vi "createSoundWave.vi"(7 "Device ID":u32, 8 "error in (no error)":errorcluster, 9 "duration (s)":dbl, 10 "frequency":dbl=10.0 format="%0.2p", 11 "Volume":dbl(slide)=50.0 scale=0.0..100.0) -> (0 "error out":errorcluster, 3 "Sound out":refnum<class "Sound.lvclass">)   [LabVIEW 2019, in "Sound.lvclass"]
uses:
  Sound.lvclass
  <vilib>/sound2/lvsound2.llb/Sampling Mode.ctl
  <vilib>/sound2/lvsound2.llb/Sound Data Format.ctl
  Sound.lvclass/Sound.ctl
  <vilib>/sound2/lvsound2.llb/Sound Output Set Volume (Single).vi
  <vilib>/measure/NI_MABase.lvlib
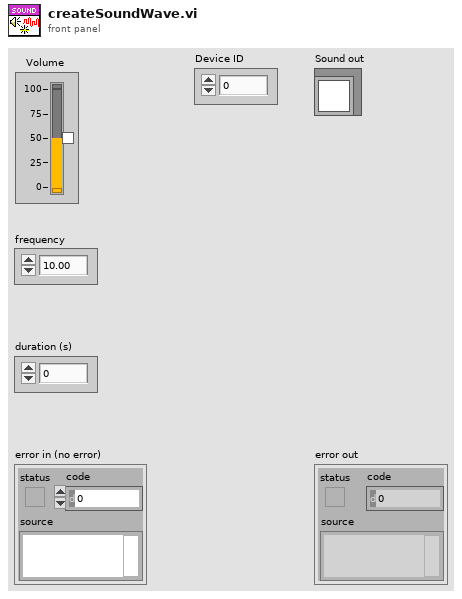
[diagram p1: front panel]
types:
  T1 = typedef "Sound Data Format.ctl" = cluster{"sample rate (S/s)":dbl, "number of channels":i32, "bits per sample":i32}
  T2 = typedef "Sampling Mode.ctl" = i32
  T3 = typedef "Sound Output Task ID.ctl" = u32
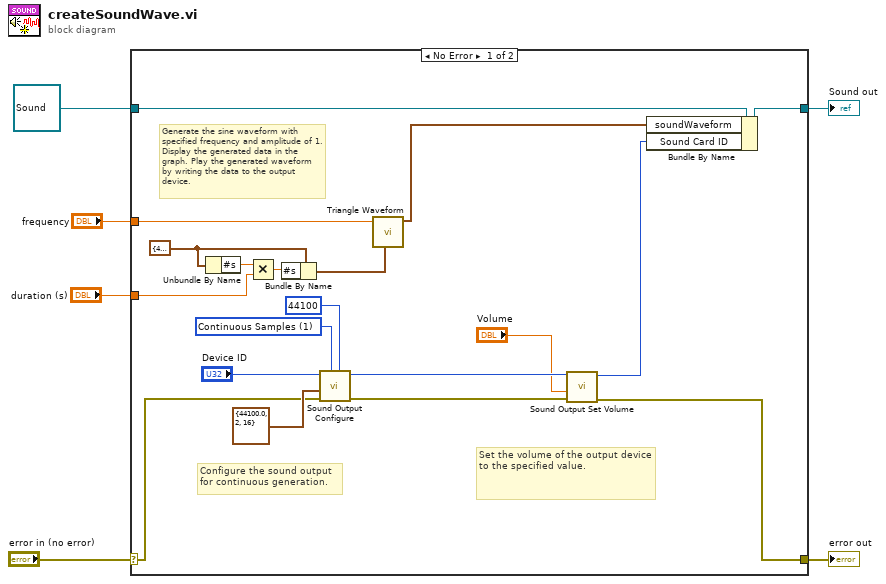
[diagram p0: block diagram]
diagram:
  n1 = case shown="No Error" "error in (no error)" {
    selector: "error in (no error)" -> [w8 w27]
    tunnel: [w7 w27] -> w5
    tunnel: [w18 w26] -> w3
    tunnel: refnum<class "Sound.lvclass"> refnum ("Sound in") -> [w25 w26]
    tunnel: "frequency" -> [w24 _]
    tunnel: "duration (s)" -> [w20 _]
    frame No Error {
      w13 = T2 1 items=["Finite Samples", "Continuous Samples"] ("sample mode")
      w22 = cluster{"Fs":dbl, "#s":dbl} {"Fs"=44100.0, "#s"=44100.0} ("sampling info")
      # "Generate the sine waveform with specified frequency and amplitude of 1. Display the generated data in the graph. Play the generated waveform by writing the data to the output device."
      # "Set the volume of the output device to the specified value."
      # "Configure the sound output for continuous generation."
      n2 = Unbundle By Name(w22) -> ("#s"=w23:dbl)
      n3 = Multiply(x=w23, y=w20) -> (x*y=w21:dbl)
      n4 = Bundle By Name(cluster=w22, "#s"=w21) -> (w19:cluster{"Fs":dbl, "#s":dbl})
      n5 = call <vilib>:"Sound Output Configure.vi"("number of samples/ch"=44100 ("Number of Samples/ch"), "sample mode"=w13, "error in (no error)"=w8, "sound format"=T1 {"sample rate (S/s)"=44100.0, "number of channels"=2, "bits per sample"=16} ("Sound Format"), "device ID"="Device ID") -> ("error out"=w16:errorcluster, "task ID"=w15:T3)  [unwired: 5 in]
      n6 = call <vilib>:"Triangle Waveform.vi"("sampling info"=w19, "frequency"=w24) -> ("signal out"=w17:waveform(dbl))  [unwired: 8 in, 1 out]
      n7 = call-poly <vilib>:"Sound Output Set Volume.vi"("error in (no error)"=w16, "volume"="Volume", "task ID"=w15) -> ("error out"=w7:errorcluster, "task ID out"=w9:T3)  [unwired: 7 in]
      n8 = Bundle By Name(cluster=w25, "soundWaveform"=w17, "Sound Card ID"=w9) -> (w18:refnum<class "Sound.lvclass">)
    }
    frame Error {
    }
  }
  "error out" <- w5
  "Sound out" <- w3
